vi "axex_select_sheet.vi"(7 "activate sheet (False)":bool, 8 "error in":errorcluster, 9 "sheet name (none)":string, 10 "sheet id":i32, 11 "AX Excel instance in":T1) -> (0 "error out":errorcluster, 1 "sheet name out":string, 2 "sheet id out":i32, 3 "AX Excel instance out":T1)   [LabVIEW 2020, in "AX Excel.lvlib"]
doc: "Call this to select given sheet within given excel file. You can select the sheet either by its name string or ID (0, 1, ..., N-1). Option 'activate sheet' will select the sheet tab in the in the Excel sheet selection tab control."
uses:
  AX Excel.lvlib
  axex_instance.ctl
  <vilib>/Utility/error.llb/Error Cluster From Error Code.vi
  <vilib>/ErrorRing/Error Ring.xnode
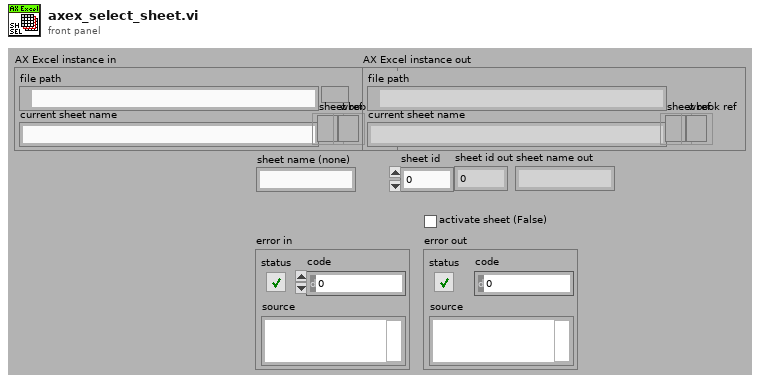
[diagram p1: front panel]
types:
  T1 = typedef "AX Excel.lvlib/axex_instance.ctl" = cluster{"file path":path, "current sheet name":string, "sheet ref":refnum<k7>, "wbook ref":refnum<k7>}
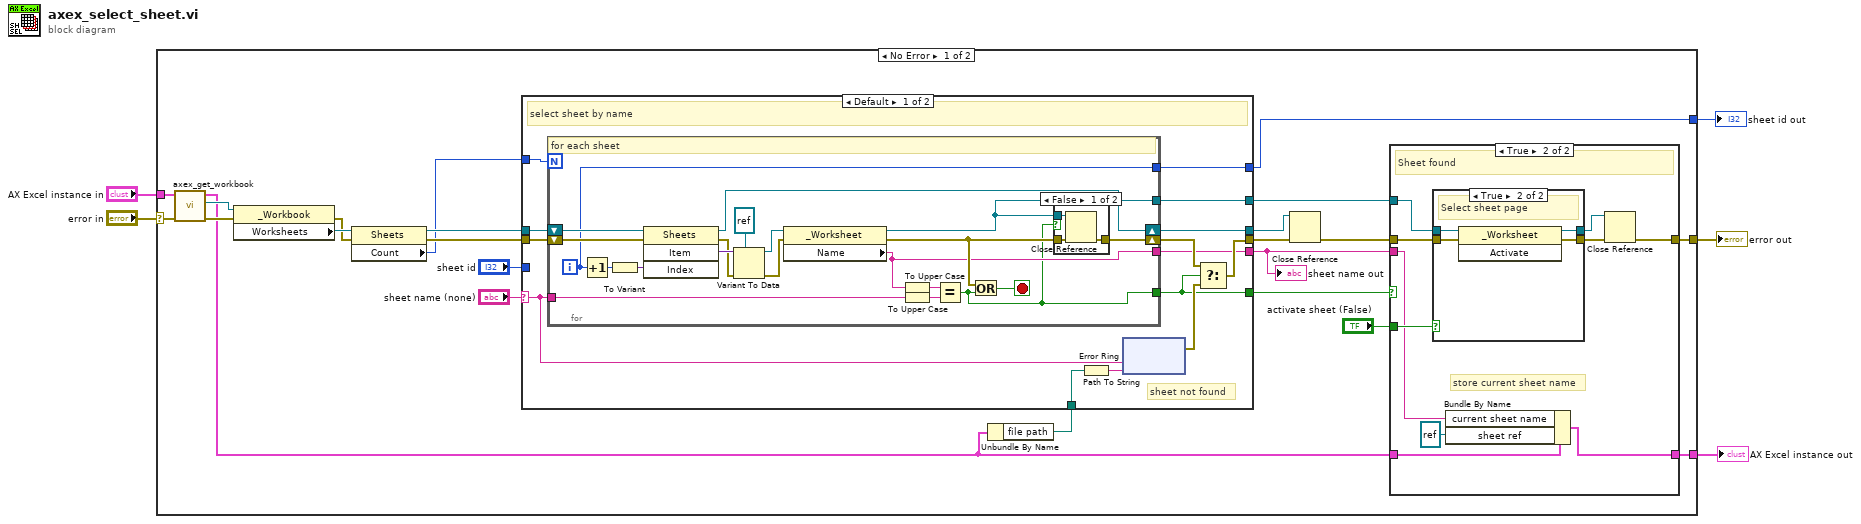
[diagram p0: block diagram]
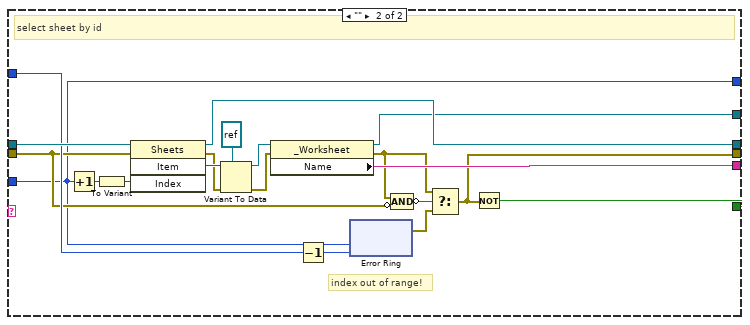
[diagram p5: hidden frame]
diagram:
  n1 = case shown="No Error" "error in" {
    selector: "error in" -> [w7 w122]
    tunnel: [w17 w122] -> w5
    tunnel: "AX Excel instance in" -> [w16 w121]
    tunnel: [w10 w121] -> w3
    tunnel: [w6 _] -> w1
    frame No Error {
      n2 = call "axex_get_workbook.vi"("error in"=w7, "AX Excel instance in"=w16) -> ("error out"=w28:errorcluster, "excel workbook"=w15:refnum<k7>, "AX Excel instance out"=w11:T1)  [unwired: 7 in]
      n3 = property class="_Workbook"(reference=w15, error in=w28) -> (error out=w26:errorcluster, "Worksheets"=w27:refnum<k7>)  [unwired: 1 out]
      n4 = property class="Sheets"(reference=w27, error in=w26) -> (reference out=w25:refnum<k7>, error out=w24:errorcluster, "Count"=w23:i32)
      n5 = Unbundle By Name(w11) -> ("file path"=w13:path)
      n6 = case shown="Default" "sheet name (none)" {
        selector: "sheet name (none)" -> [w52 _]
        tunnel: w25 -> [w60 w112]
        tunnel: w24 -> [w59 w98]
        tunnel: w23 -> [w58 w100]
        tunnel: [w53 w95] -> w22
        tunnel: [w57 w111] -> w14
        tunnel: "sheet id" -> [_ w93]
        tunnel: [w48 w102] -> w19
        tunnel: [w56 w103] -> w18
        tunnel: w13 -> [w51 _]
        tunnel: [w49 w99] -> w9
        tunnel: [w47 w93] -> w6
        frame Default {
          # "sheet not found"
          # "select sheet by name"
          n7 = for {
            N: w58 -> [_]
            shift-right: [w77] -> w54
            shift-left: w59 -> [w86]
            shift-right: [w80] -> w57
            shift-left: w60 -> [w81]
            tunnel: w52 -> [w78]
            tunnel: [w72] -> w48
            tunnel: [w75] -> w56
            tunnel: [w73] -> w49
            tunnel: [w69] -> w47
            i -> [w69]
            stop <- w74 stop-if-true
            # "for each sheet"
            n8 = Increment(x=w69) -> (x+1=w87:i32)
            n9 = To Variant(anything=w87) -> (Variant=w88:variant)
            n10 = invoke class="Sheets" method="Item"(reference=w81, error in=w86, "Index"=w88) -> (reference out=w80:refnum<k7>, error out=w83:errorcluster, "Item"=w85:variant)  [unwired: 1 in, 1 out]
            n11 = Variant To Data(error in=w83, type=refnum<k7> refnum ("reference out"), Variant=w85) -> (data=w79:refnum<k7>, error out=w82:errorcluster)
            n12 = property class="_Worksheet"(reference=w79, error in=w82) -> (reference out=w75:refnum<k7>, error out=w76:errorcluster, "Name"=w73:string)
            n13 = To Upper Case(1:w73) -> (0:w71:string)
            n14 = To Upper Case(1:w78) -> (0:w70:string)
            n15 = Equal?(x=w71, y=w70) -> (x = y?=w72:bool)
            n16 = Or(x=w76, y=w72) -> (x .or. y?=w74:bool)
            n17 = case shown="False" w72 {
              tunnel: [w91 w92] -> w77
              tunnel: w76 -> [w90 w92]
              tunnel: w75 -> [w89 _]
              frame False {
                n18 = Close Reference(reference=w89, error in (no error)=w90) -> (error out=w91:errorcluster)
              }
              frame True {
              }
            }
          }
          n19 = Path To String(path=w51) -> (string=w50:string)
          n20 = xnode "Error Ring"("parameter 0"=w52, "parameter 1"=w50) -> ("error out"=w55:errorcluster)
          n21 = Select(t=w54, s=w48, f=w55) -> (s? t:f=w53:errorcluster)
        }
        frame "" {
          # "index out of range!"
          # "select sheet by id"
          n22 = Increment(x=w93) -> (x+1=w109:i32)
          n23 = To Variant(anything=w109) -> (Variant=w110:variant)
          n24 = invoke class="Sheets" method="Item"(reference=w112, error in=w98, "Index"=w110) -> (reference out=w111:refnum<k7>, error out=w106:errorcluster, "Item"=w108:variant)  [unwired: 1 in, 1 out]
          n25 = Variant To Data(error in=w106, type=refnum<k7> refnum ("reference out"), Variant=w108) -> (data=w104:refnum<k7>, error out=w105:errorcluster)
          n26 = property class="_Worksheet"(reference=w104, error in=w105) -> (reference out=w103:refnum<k7>, error out=w96:errorcluster, "Name"=w99:string)
          n27 = Decrement(x=w100) -> (x-1=w94:i32)
          n28 = xnode "Error Ring"("parameter 0"=w93, "parameter 1"=w94) -> ("error out"=w97:errorcluster)
          n29 = Compound Arithmetic op=AND(w96, invert w98) -> (invert w101:bool)
          n30 = Select(t=w96, s=w101, f=w97) -> (s? t:f=w95:errorcluster)
          n31 = Not(x=w95) -> (.not. x?=w102:bool)
        }
      }
      "sheet name out" <- w9
      n32 = Close Reference(reference=w14, error in (no error)=w22) -> (error out=w8:errorcluster)
      n33 = case shown="True" w19 {
        tunnel: w8 -> [w30 w40]
        tunnel: w18 -> [_ w39]
        tunnel: [w30 w38] -> w17
        tunnel: "activate sheet (False)" -> [_ w37]
        tunnel: [w29 w35] -> w10
        tunnel: w11 -> [w29 w36]
        tunnel: w9 -> [_ w34]
        frame False {
        }
        frame True {
          # "store current sheet name"
          # "Sheet found"
          n34 = case shown="True" w37 {
            tunnel: w40 -> [w42 w46]
            tunnel: w39 -> [w41 w45]
            tunnel: [w41 w44] -> w32
            tunnel: [w42 w43] -> w33
            frame False {
            }
            frame True {
              # "Select sheet page"
              n35 = invoke class="_Worksheet" method="Activate"(reference=w45, error in=w46) -> (reference out=w44:refnum<k7>, error out=w43:errorcluster)  [unwired: 1 in, 1 out]
            }
          }
          n36 = Bundle By Name(cluster=w36, "current sheet name"=w34, "sheet ref"=refnum<k7> refnum) -> (w35:T1)
          n37 = Close Reference(reference=w32, error in (no error)=w33) -> (error out=w38:errorcluster)
        }
      }
    }
    frame Error {
    }
  }
  "error out" <- w5
  "AX Excel instance out" <- w3
  "sheet id out" <- w1
